vi "Test_retrigger_on_odd.vi"() -> ()   [LabVIEW 2018, in "ScopePlugins.lvlib" / "NIScope.lvclass"]
uses:
  NIScope.lvclass
  TypeDefs/Channel.ctl
  TypeDefs/Acquisition.ctl
  <instrlib>/niScope/Controls/niScope trigger slope.ctl
  <instrlib>/niScope/Controls/niScope acquisition type.ctl
  <instrlib>/niScope/Configure/Trigger/niScope Configure Trigger Digital.vi
  <instrlib>/niScope/Acquire/Fetch/niScope Multi Fetch Cluster.vi
  <instrlib>/niScope/Acquire/niScope Multi Read Cluster.vi
  ScopePlugins.lvlib
panel:
  out "wfm info":T1(array[cluster])
  out "Array":dbl[](array[numeric])
  out "x != 0?":bool
  out "time":dbl
  out "Sessions":refnum<k20>[](array[refnum])
  out "Fetch:Records Done":i32
  out "transposed array":dbl[][](array[numeric])
  out "wfm":dbl[][](array[numeric])
  out "Waveform Chart 2":dbl[][](graph)
  in  "Stop Button":bool
  out "Waveform Chart":waveform(dbl)[](graph)
  in  "Trigger":T2={"Coupling"=enum."DC", "Holdoff"=0.0, "Level"=0.2, "Slope"=enum."Positive", "Source"="PXI_Trig0", "Type"=enum."Edge"}
  in  "Acquisition":T3={"StartTime"=0.0, "Type"=enum."Normal", "NumPointsMin"=50000, "RecordLength"=50000, "SampleRate"=50000.0, "TimePerRecord"=0.001, "SamplingMode "=enum."Real Time", "Interpolation"=enum."No Interpolation", "NumAverages"=8, "Resolution"=enum."Auto", "EnableAveraging"=FALSE, "Continuous"=TRUE}
  out "error out":errorcluster
  in  "Channels":T4[](array[typedef])=[{"Enabled"=TRUE, "Name"="0", "InputImpedance"=1000000.0, "InputFreqMax"=0.0, "ProbeAttn"=1.0, "Coupling"=enum."DC", "Offset"=0.0, "Range"=10.0, "Handle"="PXI1Slot8", "Connected"=FALSE}, {"Enabled"=TRUE, "Name"="0", "InputImpedance"=1000000.0, "InputFreqMax"=0.0, "ProbeAttn"=1.0, "Coupling"=enum."DC", "Offset"=0.0, "Range"=10.0, "Handle"="PXI1Slot7", "Connected"=FALSE}, {"Enabled"=TRUE, "Name"="1", "InputImpedance"=1000000.0, "InputFreqMax"=0.0, "ProbeAttn"=1.0, "Coupling"=enum."DC", "Offset"=0.0, "Range"=10.0, "Handle"="PXI1Slot8", "Connected"=FALSE}]
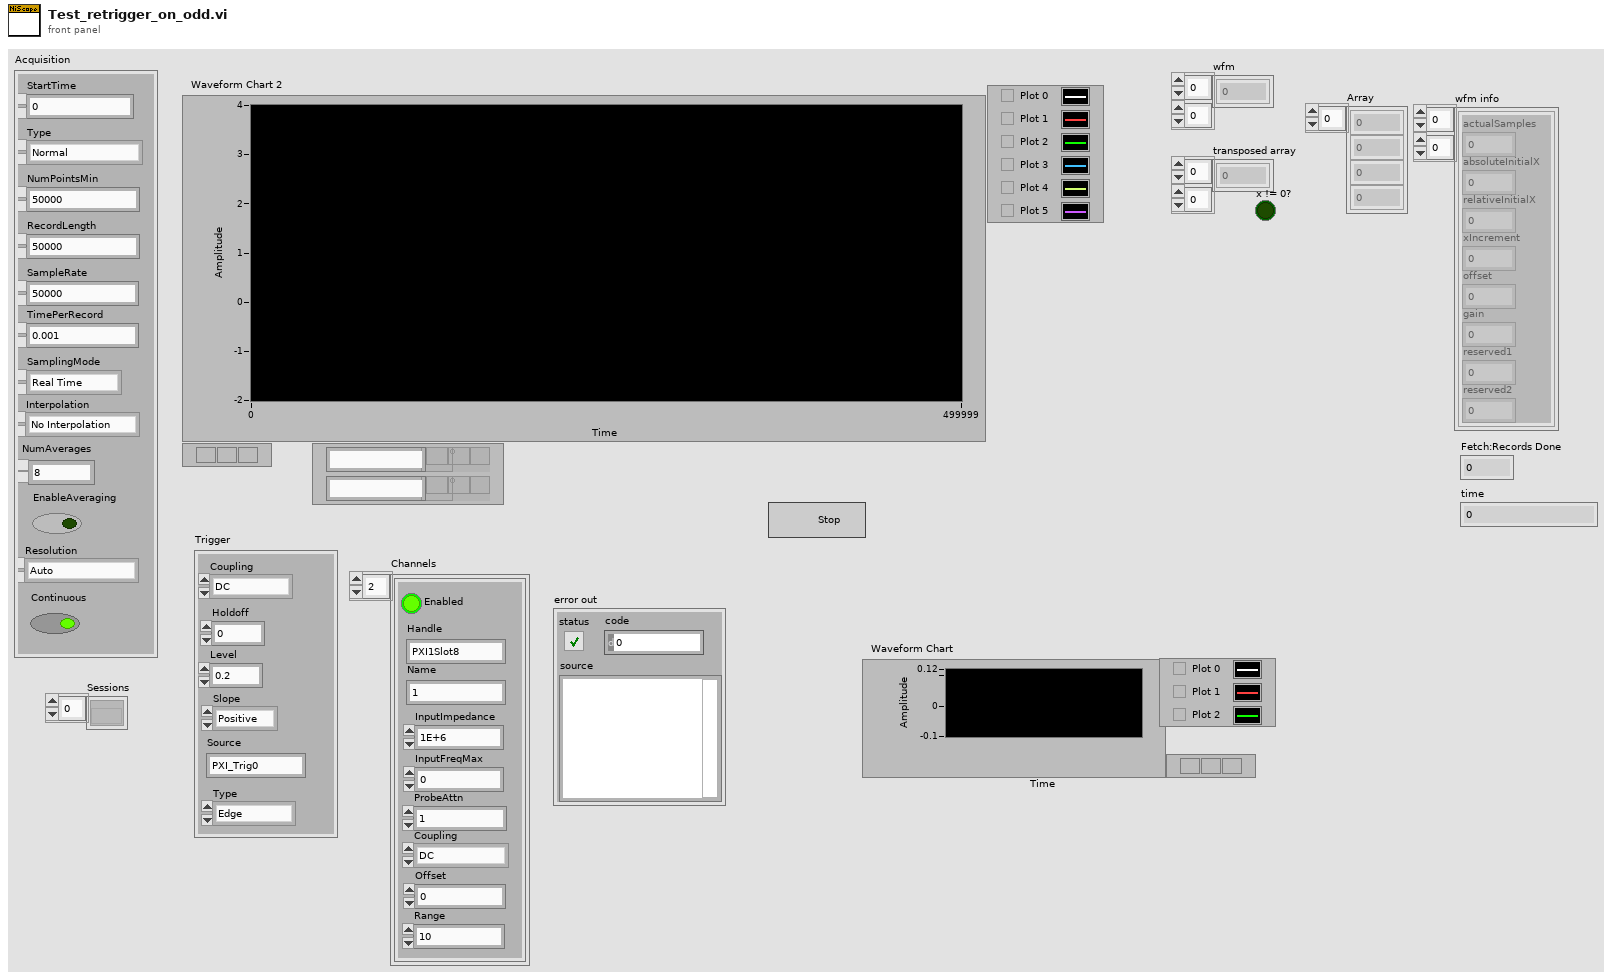
[diagram p1: front panel]
types:
  T1 = cluster{"actualSamples":i32, "absoluteInitialX":dbl, "relativeInitialX":dbl, "xIncrement":dbl, "offset":dbl, "gain":dbl, "reserved1":dbl, "reserved2":dbl}[][]
  T2 = cluster{"Coupling":enum16{"AC", "DC", "LF Reject", "HF Reject", "Noise Reject"}, "Holdoff":dbl, "Level":dbl, "Slope":enum16{"Negative", "Positive"}, "Source":string, "Type":enum16{"Edge", "Width", "Runt", "Glitch", "TV", "Immediate", "AC Line"}}
  T3 = typedef "ScopePlugins.lvlib/Acquisition.ctl" = cluster{"StartTime":dbl, "Type":enum16{"Normal", "PeakDetect", "HighRes", "Envelope", "Average"}, "NumPointsMin":i32, "RecordLength":i32, "SampleRate":dbl, "TimePerRecord":dbl, "SamplingMode ":enum16{"Real Time", "Equivalent Time", "Segment", "Real Time Peak Detect", "Real Time High Resolution", "Peak Detect Segment", "High Resolution Segment"}, "Interpolation":enum16{"No Interpolation", "sin(x)/x", "linear", "1 Point sin(x)/x", "2 Point sin(x)/x", "4 Point sin(x)/x", "8 Point sin(x)/x", "16 Point sin(x)/x"}, "NumAverages":i32, "Resolution":enum16{"Auto", "Bits 9", "Bits 10", "Bits 11", "Bits 12"}, "EnableAveraging":bool, "Continuous":bool}
  T4 = typedef "ScopePlugins.lvlib/Channel.ctl" = cluster{"Enabled":bool, "Name":string, "InputImpedance":dbl, "InputFreqMax":dbl, "ProbeAttn":dbl, "Coupling":enum16{"AC", "DC", "GND"}, "Offset":dbl, "Range":dbl, "Handle":string, "Connected":bool}
  T5 = enum16{"Normal", "PeakDetect", "HighRes", "Envelope", "Average"}
  T6 = enum16{"Real Time", "Equivalent Time", "Segment", "Real Time Peak Detect", "Real Time High Resolution", "Peak Detect Segment", "High Resolution Segment"}
  T7 = typedef "niScope acquisition type.ctl" = i32
  T8 = typedef "niScope trigger slope.ctl" = i32
  T9 = cluster{"relativeInitialX":dbl, "xIncrement":dbl, "wfm":dbl[]}[]
  T10 = cluster{"actualSamples":i32, "absoluteInitialX":dbl, "relativeInitialX":dbl, "xIncrement":dbl, "offset":dbl, "gain":dbl, "reserved1":dbl, "reserved2":dbl}[]
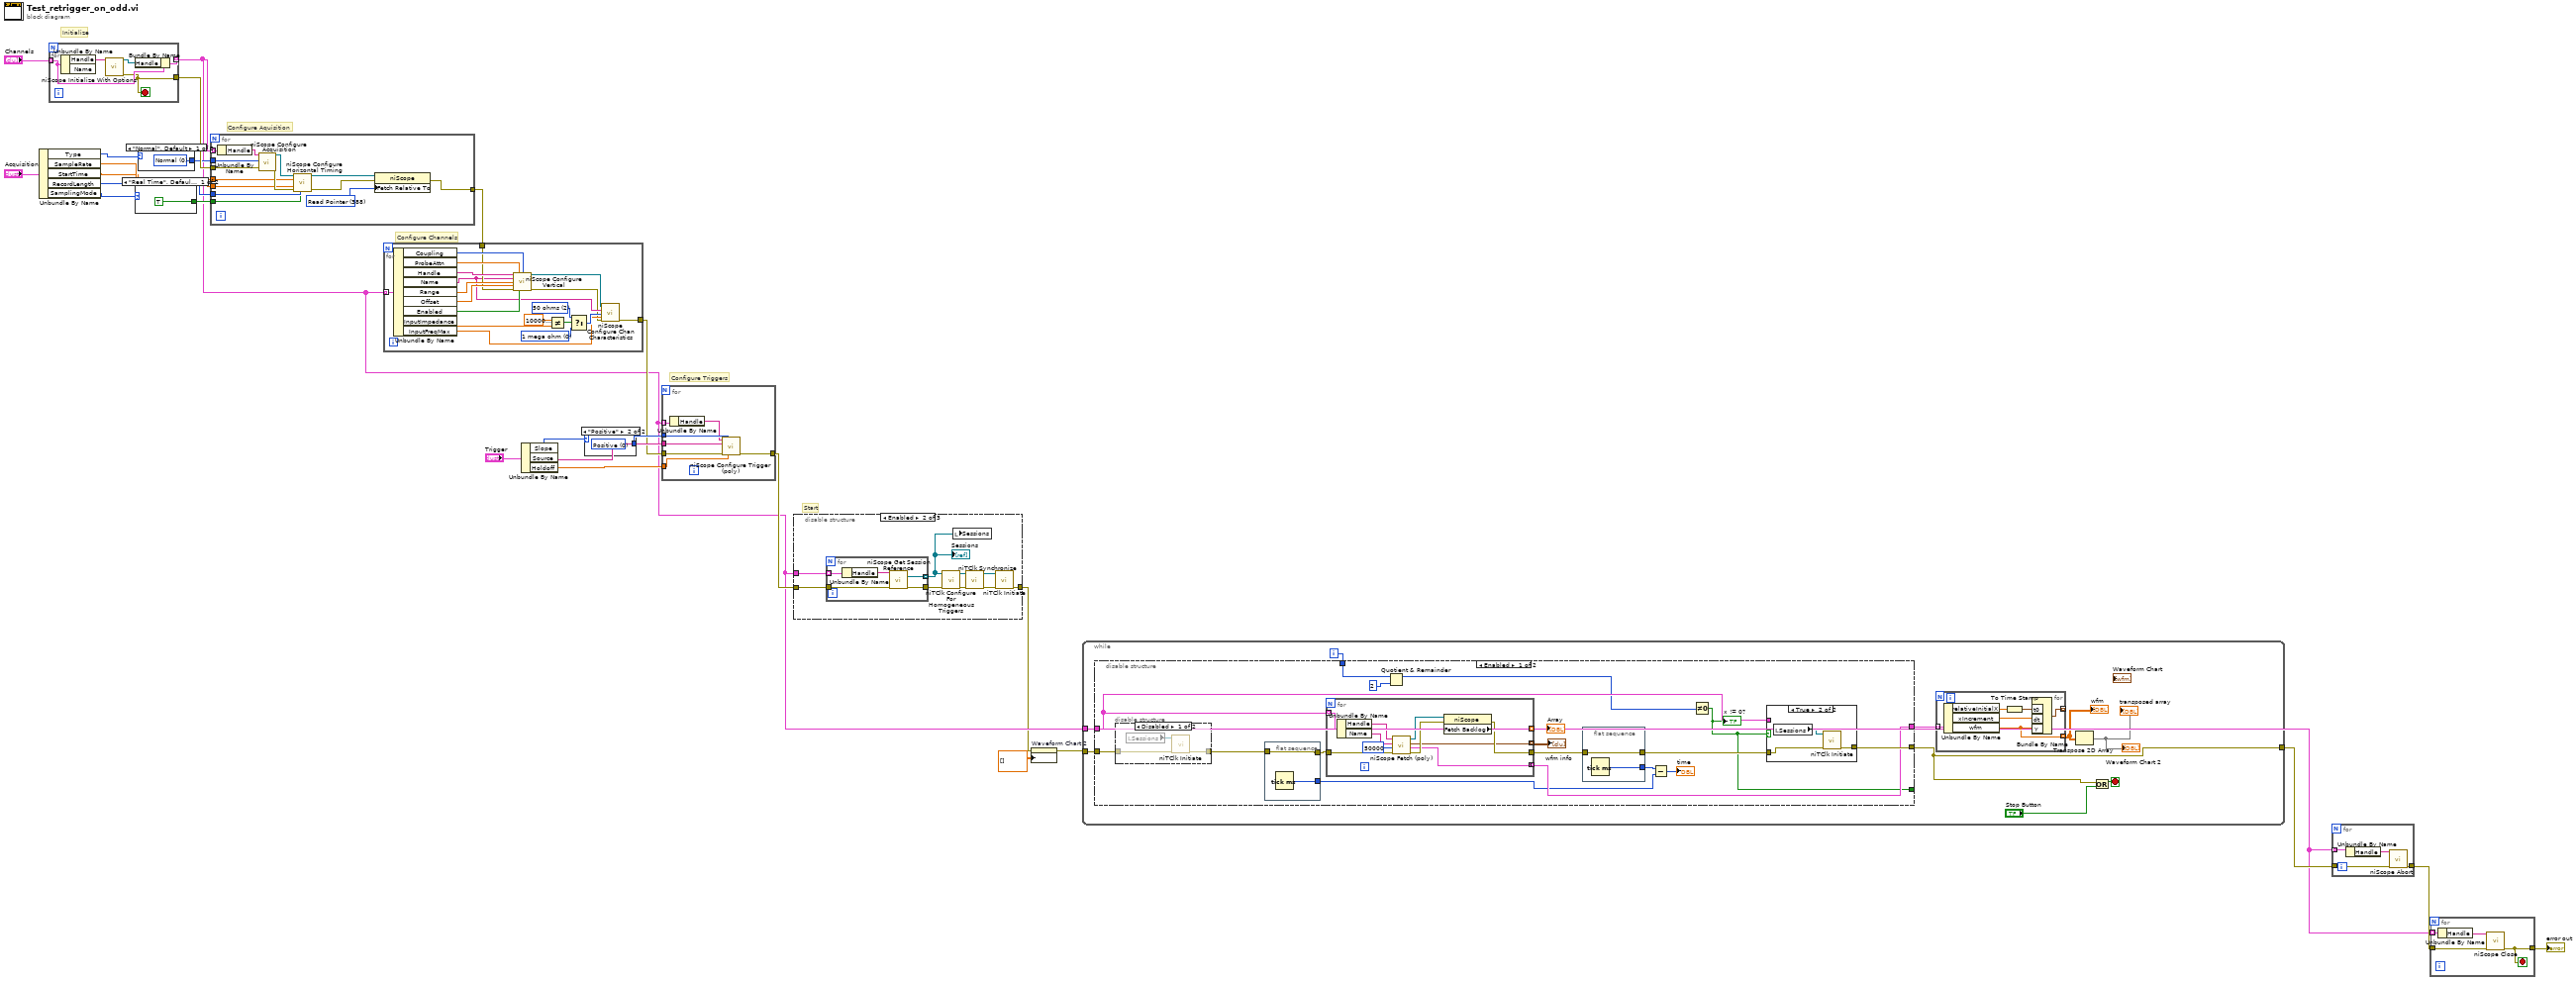
[diagram p0: block diagram]
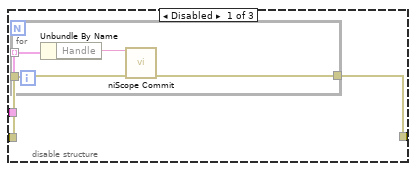
[diagram p2: hidden frame]
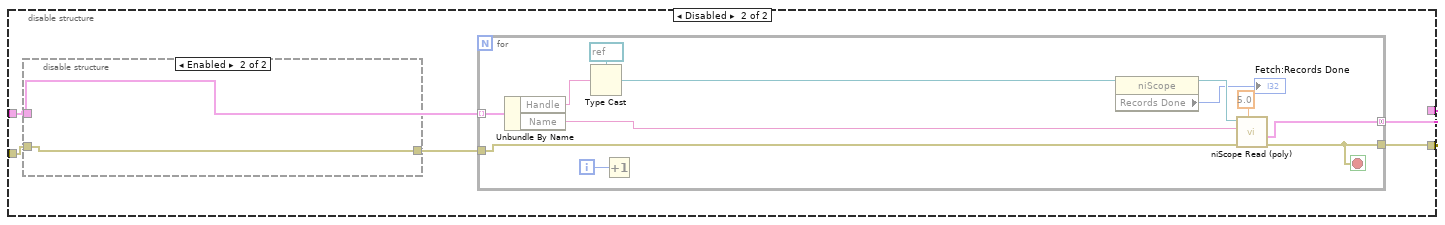
[diagram p6: hidden frame]
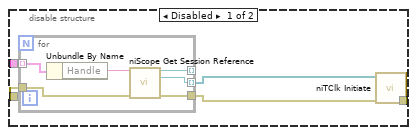
[diagram p7: hidden frame]
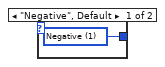
[diagram p8: hidden frame]
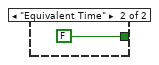
[diagram p9: hidden frame]
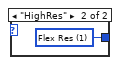
[diagram p10: hidden frame]
diagram:
  # "Start"
  # "Configure Triggers"
  # "Configure Channels"
  # "Configure Aquisition"
  # "Initialize"
  n1 = Unbundle By Name("Acquisition") -> ("Type"=w22:T5, "SampleRate"=w18:dbl, "StartTime"=w17:dbl, "RecordLength"=w16:i32, "SamplingMode"=w21:T6)
  n2 = for {
    tunnel: "Channels" -> [w29] mode=indexing
    tunnel: [w26] -> w20
    tunnel: [w28] -> w4 mode=indexing
    stop <- w26 stop-if-true
    n3 = Unbundle By Name(w29) -> ("Handle"=w30:string)  [unwired: 1 out]
    n4 = call <instrlib>:"niScope Initialize With Options.vi"("resource name"=w30) -> ("instrument handle"=w27:refnum<k15>, "error out"=w26:errorcluster)  [unwired: 13 in]
    n5 = Bundle By Name(cluster=w29, "Handle"=w27) -> (w28:T4)
  }
  n6 = case shown="\"Real Time\", Default" w21 {
    tunnel: [TRUE FALSE] -> w9
    frame "Real Time", Default {
    }
    frame "Equivalent Time" {
    }
  }
  n7 = case shown="\"Normal\", Default" w22 {
    tunnel: [w33 w34] -> w19
    frame "Normal", Default {
      w33 = T7 0 items=["Normal"=0, "Flex Res"=1, "DDC"=3] ("acquisition Type")
    }
    frame "HighRes" {
      w34 = T7 1 items=["Normal"=0, "Flex Res"=1, "DDC"=3] ("acquisition Type")
    }
  }
  n8 = for {
    tunnel: w4 -> [w47] mode=indexing
    tunnel: w20 -> [w45]
    tunnel: w19 -> [w48]
    tunnel: w18 -> [w42]
    tunnel: w17 -> [w41]
    tunnel: w16 -> [w40]
    tunnel: [w37] -> w10
    tunnel: w9 -> [w38]
    w35 = 388 items=["Start"=482, "Trigger"=483, "Pretrigger"=477, "Now"=481, "Read Pointer"=388] ("Fetch:Fetch Relative To")
    n9 = Unbundle By Name(w47) -> ("Handle"=w46:string)
    n10 = call <instrlib>:"niScope Configure Acquisition.vi"("instrument handle"=w46, "acquisition Type"=w48, "error in"=w45) -> ("instrument handle out"=w44:refnum<k15>, "error out"=w43:errorcluster)  [unwired: 11 in]
    n11 = call <instrlib>:"niScope Configure Horizontal Timing.vi"("instrument handle"=w44, "enforce realtime"=w38, "min sample rate"=w42, "reference position"=w41, "error in"=w43, "min record length"=w40) -> ("instrument handle out"=w36:refnum<k15>, "error out"=w39:errorcluster)  [unwired: 8 in]
    n12 = property class="niScope"(reference=w36, error in=w39, "Fetch Relative To"=w35) -> (error out=w37:errorcluster)  [unwired: 1 out]
  }
  n13 = for {
    tunnel: w4 -> [w67] mode=indexing
    tunnel: w10 -> [w61]
    tunnel: [w50] -> w8
    w59 = u32 0 items=["1 mega ohm"=0, "50 ohms"=2] ("input impedance")
    w54 = u32 2 items=["1 mega ohm"=0, "50 ohms"=2] ("input impedance")
    n14 = Unbundle By Name(w67) -> ("Coupling"=w66:enum16{"AC", "DC", "GND"}, "ProbeAttn"=w65:dbl, "Handle"=w64:string, "Name"=w52:string, "Range"=w63:dbl, "Offset"=w62:dbl, "Enabled"=w60:bool, "InputImpedance"=w55:dbl, "InputFreqMax"=w53:dbl)
    n15 = call <instrlib>:"niScope Configure Vertical.vi"("instrument handle"=w64, "probe attenuation"=w65, "vertical coupling"=w66, "channels"=w52, "vertical range"=w63, "vertical offset"=w62, "error in"=w61, "channel enabled"=w60) -> ("instrument handle out"=w49:refnum<k15>, "error out"=w51:errorcluster)  [unwired: 6 in]
    n16 = Not Equal?(x=1000000.0, y=w55) -> (x != y?=w57:bool)
    n17 = Select(t=w54, s=w57, f=w59) -> (s? t:f=w56:u32)
    n18 = call <instrlib>:"niScope Configure Chan Characteristics.vi"("instrument handle"=w49, "channels"=w52, "input impedance"=w56, "maximum input frequency"=w53, "error in"=w51) -> ("error out"=w50:errorcluster)  [unwired: 9 in, 1 out]
  }
  n19 = Unbundle By Name("Trigger") -> ("Slope"=w14:enum16{"Negative", "Positive"}, "Source"=w12:string, "Holdoff"=w11:dbl)
  n20 = case shown="\"Positive\"" w14 {
    tunnel: [w68 w69] -> w13
    frame "Negative", Default {
      w68 = T8 1 items=["Positive", "Negative"] ("trigger slope")
    }
    frame "Positive" {
      w69 = T8 0 items=["Positive", "Negative"] ("trigger slope")
    }
  }
  n21 = for {
    tunnel: w13 -> [w76]
    tunnel: w12 -> [w75]
    tunnel: w11 -> [w74]
    tunnel: w8 -> [w73]
    tunnel: [w72] -> w7
    tunnel: w4 -> [w71] mode=indexing
    n22 = Unbundle By Name(w71) -> ("Handle"=w70:string)
    n23 = call-poly <instrlib>:"niScope Configure Trigger (poly).vi"("instrument handle"=w70, "trigger slope"=w76, "trigger source"=w75, "error in"=w73, "trigger holdoff"=w74) -> ("error out"=w72:errorcluster)  [unwired: 9 in, 1 out]
  }
  n24 = disable-structure shown="Enabled" {
    disable-tunnel: w7 -> [w79 w92 w98]
    disable-tunnel: [w78 w86 w98] -> w2
    disable-tunnel: w4 -> [w77 w91 _]
    frame Disabled {
      n25 = for {
        tunnel: w77 -> [w83] mode=indexing
        tunnel: w79 -> [w81]
        tunnel: [w80] -> w78
        n26 = Unbundle By Name(w83) -> ("Handle"=w82:string)
        n27 = call <instrlib>:"niScope Commit.vi"("instrument handle"=w82, "error in"=w81) -> ("error out"=w80:errorcluster)  [unwired: 12 in, 1 out]
      }
    }
    frame Enabled {
      n28 = for {
        tunnel: [w97] -> w84 mode=indexing
        tunnel: [w96] -> w90
        tunnel: w91 -> [w95] mode=indexing
        tunnel: w92 -> [w93]
        n29 = Unbundle By Name(w95) -> ("Handle"=w94:string)
        n30 = call <instrlib>:"niScope Get Session Reference.vi"("instrument handle"=w94, "error in"=w93) -> ("session reference"=w97:refnum<k20>, "error out"=w96:errorcluster)  [unwired: 11 in, 1 out]
      }
      "Sessions" <- w84
      n31 = call <instrlib>:"niTClk Configure For Homogeneous Triggers.vi"("error in (no error)"=w90, "sessions"=w84) -> ("error out"=w89:errorcluster, "sessions out"=w88:refnum<k20>[])  [unwired: 8 in]
      n32 = local write "Sessions"(w84) -> ()
      n33 = call <instrlib>:"niTClk Synchronize.vi"("error in (no error)"=w89, "sessions"=w88) -> ("error out"=w87:errorcluster, "sessions out"=w85:refnum<k20>[])  [unwired: 8 in]
      n34 = call <instrlib>:"niTClk Initiate.vi"("error in (no error)"=w87, "sessions"=w85) -> ("error out"=w86:errorcluster)  [unwired: 8 in, 1 out]
    }
    frame Disabled {
    }
  }
  n35 = property on="Waveform Chart 2" class="WFChart (strict)"(error in=w2, "History Data"=dbl[][] []) -> (error out=w3:errorcluster)  [unwired: 1 in, 1 out]
  n36 = while {
    tunnel: w4 -> [w106]
    tunnel: w3 -> [w107]
    tunnel: [w101] -> w6
    i -> [w100]
    stop <- w102 stop-if-true
    n37 = disable-structure shown="Enabled" {
      disable-tunnel: w107 -> [w124 w150]
      disable-tunnel: [w123 w151] -> w101
      disable-tunnel: w106 -> [w121 w148]
      disable-tunnel: [w122 w152] -> w105
      disable-tunnel: w100 -> [w119 _]
      disable-tunnel: [w108 _] -> _
      frame Enabled {
        n38 = disable-structure shown="Disabled" {
          disable-tunnel: w124 -> [w133 w136]
          disable-tunnel: [w135 w136] -> w118
          frame Disabled {
            n39 = local read "Sessions"() -> (w134:refnum<k20>[])
            n40 = call <instrlib>:"niTClk Initiate.vi"("error in (no error)"=w133, "sessions"=w134) -> ("error out"=w135:errorcluster)  [unwired: 8 in, 1 out]
          }
          frame Enabled {
          }
        }
        n41 = flat-sequence {
          tunnel: w118 -> [w128]
          tunnel: [w128] -> w117
          tunnel: [w127] -> w113
          frame #0 {
            n42 = Tick Count (ms)() -> (millisecond timer value=w127:u32)
          }
        }
        n43 = for {
          tunnel: w117 -> [w147]
          tunnel: [w140] -> w116
          tunnel: [w139] -> w122 mode=concatenating
          tunnel: w121 -> [w146] mode=indexing
          tunnel: [w141] -> w111 mode=indexing
          tunnel: [w138] -> w110 mode=indexing
          n44 = Unbundle By Name(w146) -> ("Handle"=w145:string, "Name"=w144:string)
          n45 = call-poly <instrlib>:"niScope Fetch (poly).vi"("error in"=w147, "numSamples"=50000, "channels"=w144, "instrument handle"=w145) -> ("error out"=w142:errorcluster, "waveform"=w139:T9, "wfm info"=w138:T10, "instrument handle out"=w143:refnum<k15>)  [unwired: 4 in]
          n46 = property class="niScope"(reference=w143, error in=w142) -> (error out=w140:errorcluster, "Fetch Backlog"=w141:dbl)  [unwired: 1 out]
        }
        "Array" <- w111
        "wfm info" <- w110
        n47 = Quotient & Remainder(x=w119, y=2) -> (x-y*floor(x/y)=w109:i32)  [unwired: 1 out]
        n48 = flat-sequence {
          tunnel: w116 -> [w126]
          tunnel: [w126] -> w115
          tunnel: [w125] -> w114
          frame #0 {
            n49 = Tick Count (ms)() -> (millisecond timer value=w125:u32)
          }
        }
        n50 = Subtract(x=w114, y=w113) -> (x-y=→"time":u32)
        n51 = Not Equal To 0?(x=w109) -> (x != 0?=w108:bool)
        "x != 0?" <- w108
        n52 = case shown="True" w108 {
          tunnel: w121 -> [_ _]
          tunnel: w115 -> [w129 w130]
          tunnel: [w129 w132] -> w123
          frame False {
          }
          frame True {
            n53 = local read "Sessions"() -> (w131:refnum<k20>[])
            n54 = call <instrlib>:"niTClk Initiate.vi"("error in (no error)"=w130, "sessions"=w131) -> ("error out"=w132:errorcluster)  [unwired: 8 in, 1 out]
          }
        }
      }
      frame Disabled {
        n55 = disable-structure shown="Enabled" {
          disable-tunnel: w150 -> [w157 w164]
          disable-tunnel: w148 -> [w154 _]
          disable-tunnel: [w153 w164] -> w149
          frame Disabled {
            n56 = for {
              tunnel: [w163] -> w155 mode=indexing
              tunnel: [w162] -> _ mode=indexing
              tunnel: [w161] -> w156
              tunnel: w154 -> [w160] mode=indexing
              tunnel: w157 -> [w158]
              n57 = Unbundle By Name(w160) -> ("Handle"=w159:string)
              n58 = call <instrlib>:"niScope Get Session Reference.vi"("instrument handle"=w159, "error in"=w158) -> ("instrument handle out"=w162:refnum<k15>, "session reference"=w163:refnum<k20>, "error out"=w161:errorcluster)  [unwired: 11 in]
            }
            n59 = call <instrlib>:"niTClk Initiate.vi"("error in (no error)"=w156, "sessions"=w155) -> ("error out"=w153:errorcluster)  [unwired: 8 in, 1 out]
          }
          frame Enabled {
          }
        }
        n60 = for {
          tunnel: w148 -> [w176] mode=indexing
          tunnel: [w174] -> w151
          tunnel: [w175] -> w152 mode=concatenating
          tunnel: w149 -> [w165]
          i -> [w166]
          stop <- w174 stop-if-true
          n61 = Unbundle By Name(w176) -> ("Handle"=w170:string, "Name"=w171:string)
          n62 = Type Cast(type=refnum<k15> refnum ("instrument handle"), x=w170) -> (*(type *) &x=w169:refnum<k15>)
          n63 = Increment(x=w166) -> ()  [unwired: 1 out]
          n64 = property class="niScope"(reference=w169) -> (reference out=w168:refnum<k15>, "Records Done"=→"Fetch:Records Done":i32)  [unwired: 1 in, 1 out]
          n65 = call-poly <instrlib>:"niScope Read (poly).vi"("timeout"=5.0, "error in"=w165, "channels"=w171, "instrument handle"=w168) -> ("error out"=w174:errorcluster, "waveform"=w175:T9)  [unwired: 4 in, 2 out]
        }
      }
    }
    n66 = for {
      tunnel: w105 -> [w182] mode=indexing
      tunnel: [w178] -> _ mode=indexing
      tunnel: [w177] -> w104 mode=indexing
      n67 = Unbundle By Name(w182) -> ("relativeInitialX"=w181:dbl, "xIncrement"=w179:dbl, "wfm"=w177:dbl[])
      n68 = To Time Stamp(1:w181) -> (0:w180:timestamp)
      n69 = Bundle By Name("t0"=w180, "dt"=w179, "Y"=w177) -> (w178:waveform(dbl))  [unwired: 1 in]
    }
    "wfm" <- w104
    n70 = Transpose 2D Array(2D array=w104) -> (transposed array=→"Waveform Chart 2" →"transposed array":dbl[][])
    n71 = Or(x=w101, y="Stop Button") -> (x .or. y?=w102:bool)
  }
  n72 = for {
    tunnel: w4 -> [w186] mode=indexing
    tunnel: w6 -> [w185]
    tunnel: [w183] -> w5
    n73 = Unbundle By Name(w186) -> ("Handle"=w184:string)
    n74 = call <instrlib>:"niScope Abort.vi"("instrument handle"=w184, "error in"=w185) -> ("error out"=w183:errorcluster)  [unwired: 12 in, 1 out]
  }
  n75 = for {
    tunnel: [w190] -> w24
    tunnel: w4 -> [w188] mode=indexing
    tunnel: w5 -> [w187]
    stop <- w190 stop-if-true
    n76 = Unbundle By Name(w188) -> ("Handle"=w189:string)
    n77 = call <instrlib>:"niScope Close.vi"("instrument handle"=w189, "error in"=w187) -> ("error out"=w190:errorcluster)  [unwired: 13 in]
  }
  "error out" <- w24
